vi "Retrieve and Scale Measurement.vi"(0 "private data":T1={"GTX2_CHANNEL register map"=refnum, "instruction target"=refnum, "channel measure state"=enum."Uninitialized", "in DFE mode?"=FALSE, "prescale"=0, "rx internal data width"=enum."32 Bit", "active point"={"horizontal offset"=0, "vertical offset"=0}, "ut sign"=enum."Positive", "positive counts"={"sample count"=0, "error count"=0}, "negative counts"={"sample count"=0, "error count"=0}}, 11 "error in":errorcluster) -> (4 "private data out":T1={"GTX2_CHANNEL register map"=refnum, "instruction target"=refnum, "channel measure state"=enum."Uninitialized", "in DFE mode?"=FALSE, "prescale"=0, "rx internal data width"=enum."32 Bit", "active point"={"horizontal offset"=0, "vertical offset"=0}, "ut sign"=enum."Positive", "positive counts"={"sample count"=0, "error count"=0}, "negative counts"={"sample count"=0, "error count"=0}}, 6 "bit error ratio":dbl, 8 "sample count":u64, 10 "error count":u64, 15 "error out":errorcluster)   [LabVIEW 2015, in "niHighSpeedSerial Eye Scan Single Point v1 Host.lvclass"]
doc: "Retrieves the saved <b>sample count(s)</b> and <b>error count(s)</b>, scales the <b>sample count(s)</b>, and computes the <b>bit error rate</b>.\n\n<B>Input Parameters</B>\n\n<B>private data</B> is the class private data input into the VI.\n\n<B>private data.GTX2_CHANNEL register map</B> is the GTX2 Channel register map to use.\n\n<B>private data.instruction target</B> is the instruction target to use when communicating with the FPGA.\n\n<B>private data.channel measure state</B> maintains the internal state of the Eye Scan Single Point class.\nenum values: Uninitialized,Initialized,Ready,Request,Wait,Read,Process,Finished\n\n<B>private data.in DFE mode?</B> is true if Eye Scan is configured for DFE Equalization Mode.\n\n<B>private data.prescale</B> controls scaling of the sample count in order to keep the sample count and error count within reasonable precision.\n\n<B>private data.receiver data width</B> is the data width (in bits) of the receiver lane.\nenum values: 16 Bit,20 Bit,32 Bit,40 Bit\n\n<B>private data.active point</B> is the point currently being sampled for errors using Eye Scan.\n\n<B>private data.active point.horizontal offset</B> is the horizontal offset of the active point.\n\n<B>private data.active point.vertical offset</B> is the vertical offset of the active point.\n\n<B>private data.ut sign</B> The untapped threshold sign (positive or negative) currently configured on the point being measured.\nPositive is used when in DFE or LPM Equalization Mode, while Negative is only used in DFE Equalization Mode.\n\n<B>private data.positive counts</B> contains the number of sample and error counts measured using the positive UT Sign.\n\n<B>private data.positive counts.sample count</B> is the positive sample count when using DFE mode, or the entire sample count when using LPM mode.\n\n<B>private data.positive counts.error count</B> is the positive error count when using DFE mode, or the entire error count when using LPM mode.\n\n<B>private data.negative counts</B> contains the number of sample and error counts measured using the negative UT Sign.\n\n<B>private data.negative counts.sample count</B> is the negative sample count when using DFE mode, or unused when using LPM mode.\n\n<B>private data.negative counts.error count</B> is the negative error count when using DFE mode, or unused when using LPM mode.\n\n<B>error in</B> describes error conditions that occur before this node runs. This input provides standard 'error in' functionality.\n\n<B>Output Parameters</B>\n\n<B>private data out</B> is the class private data output from the VI.\n\n<B>private data out.GTX2_CHANNEL register map</B> is the register map to use which represents the GTX2 Channel.\n\n<B>private data out.instruction target</B> is the instruction target to use when communicating with the FPGA.\n\n<B>private data out.channel measure state</B> maintains the internal state of the Eye Scan Single Point class.\nenum values: Uninitialized,Initialized,Ready,Request,Wait,Read,Process,Finished\n\n<B>private data out.in DFE mode?</B> is true if Eye Scan is configured for DFE Equalization Mode.\n\n<B>private data out.prescale</B> controls scaling of the sample count in order to keep the sample count and error count within reasonable precision.\n\n<B>private data out.receiver data width</B> is the data width (in bits) of the receiver lane.\nenum values: 16 Bit,20 Bit,32 Bit,40 Bit\n\n<B>private data out.active point</B> is the point currently being sampled for errors using Eye Scan.\n\n<B>private data out.active point.horizontal offset</B> is the horizontal offset of the active point.\n\n<B>private data out.active point.vertical offset</B> is the vertical offset of the active point.\n\n<B>private data out.ut sign</B> contains the number of sample and error counts measured using the positive UT Sign.\nenum values: Positive,Negative\n\n<B>private data out.positive counts</B> contains the number of sample and error counts measured using the positive UT Sign.\n\n<B>private data out.positive counts.sample count</B> is the positive sample count when using DFE mode, or the entire sample count when using LPM mode.\n\n<B>private data out.positive counts.error count</B> is the positive error count when using DFE mode, or the entire error count when using LPM mode.\n\n<B>private data out.negative counts</B> contains the number of sample and error counts measured using the negative UT Sign.\n\n<B>private data out.negative counts.sample count</B> is the negative sample count when using DFE mode, or the entire sample count when using LPM mode.\n\n<B>private data out.negative counts.error count</B> is the negative error count when using DFE mode, or the entire error count when using LPM mode.\n\n<B>bit error rate</B> is the calculated statistical bit error rate based on the number of error counts and sample counts received.\n\n<B>sample count</B> is the number of samples that have been measured on this point.\n\n<B>error count</B> is the number of errors that have been measured on this point.\n\n<B>error out</B> contains error information. This output provides standard 'error out' functionality."
uses:
  <instrlib>/niHighSpeedSerial/Eye Scan/v1/Host/Impl/Single Point/niHighSpeedSerial Eye Scan Single Point v1 Host.lvclass
  <instrlib>/niHighSpeedSerial/Eye Scan/v1/Host/Impl/Single Point/Private/Private Data.ctl
  <instrlib>/niHighSpeedSerial/Register Maps/Xilinx/v1/Host/GTX2_CHANNEL v1 Host.llb/GTX2_CHANNEL Register Map.lvclass
  <instrlib>/_niInstr/Instruction Framework/v1/Host/Instruction Target/niInstr Instruction Target v1 Host.lvclass
  <instrlib>/niHighSpeedSerial/Eye Scan/v1/Host/Impl/Single Point/Private/Channel Measure State.ctl
  <instrlib>/niHighSpeedSerial/Eye Scan/v1/Host/Common/Public/Data Width.ctl
  <instrlib>/niHighSpeedSerial/Eye Scan/v1/Host/Common/Public/Point Offsets.ctl
  <instrlib>/niHighSpeedSerial/Register Maps/Xilinx/v1/Host/GTX2_CHANNEL v1 Host.llb/ESVertOffsetSign.ctl
  <instrlib>/niHighSpeedSerial/Eye Scan/v1/Host/Impl/Single Point/Private/Counts.ctl
  <instrlib>/niHighSpeedSerial/Eye Scan/v1/Host/Common/niHighSpeedSerial Eye Scan Common v1 Host.lvlib
  <instrlib>/niHighSpeedSerial/Register Maps/Xilinx/v1/Host/GTX2_CHANNEL v1 Host.llb/GTX2_CHANNEL v1 Host.lvlib
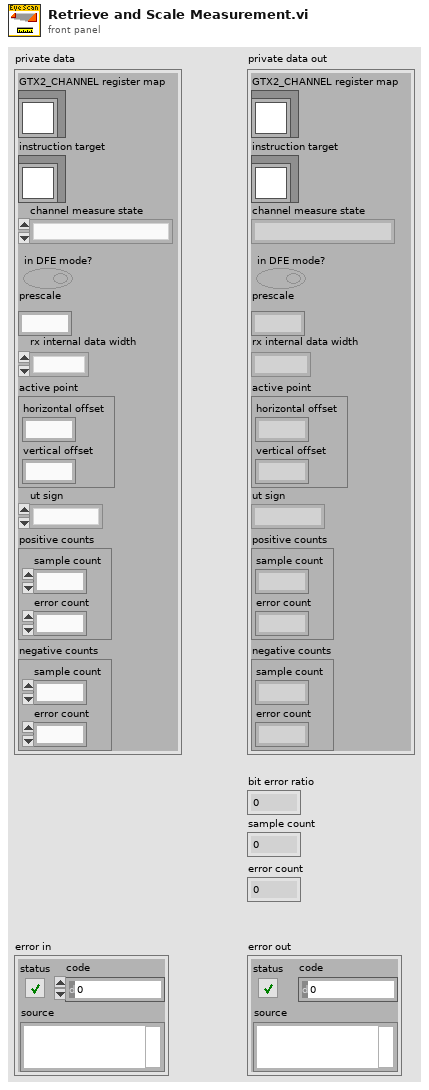
[diagram p1: front panel]
types:
  T1 = typedef "niHighSpeedSerial Eye Scan Single Point v1 Host.lvclass/Private Data.ctl" = cluster{"GTX2_CHANNEL register map":refnum<class "GTX2_CHANNEL Register Map.lvclass">, "instruction target":refnum<class "niInstr Instruction Target v1 Host.lvclass">, "channel measure state":T2, "in DFE mode?":bool, "prescale":u8, "rx internal data width":T3, "active point":T4, "ut sign":T5, "positive counts":T6, "negative counts":T6}
  T2 = typedef "niHighSpeedSerial Eye Scan Single Point v1 Host.lvclass/Channel Measure State.ctl" = enum16{"Uninitialized", "Initialized", "Ready", "Request", "Wait", "Read", "Process", "Finished"}
  T3 = typedef "niHighSpeedSerial Eye Scan Common v1 Host.lvlib/Data Width.ctl" = enum16{"16 Bit", "20 Bit", "32 Bit", "40 Bit"}
  T4 = typedef "niHighSpeedSerial Eye Scan Common v1 Host.lvlib/Point Offsets.ctl" = cluster{"horizontal offset":i16, "vertical offset":i8}
  T5 = typedef "GTX2_CHANNEL v1 Host.lvlib/ESVertOffsetSign.ctl" = enum8{"Positive", "Negative"}
  T6 = typedef "niHighSpeedSerial Eye Scan Single Point v1 Host.lvclass/Counts.ctl" = cluster{"sample count":u64, "error count":u16}
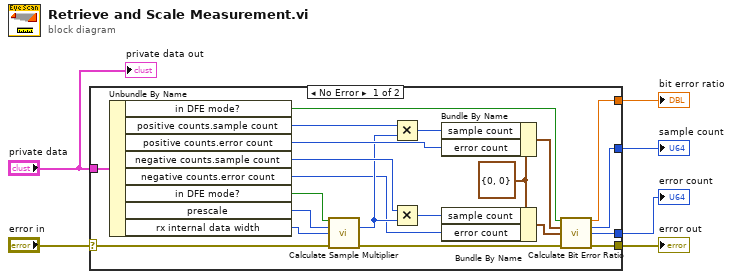
[diagram p0: block diagram]
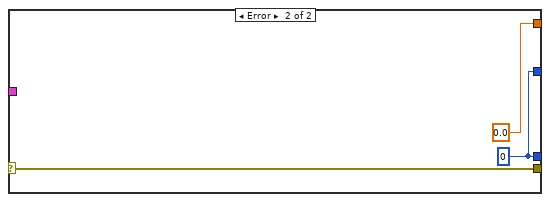
[diagram p2: hidden frame]
diagram:
  n1 = case shown="No Error" "error in" {
    selector: "error in" -> [w27 w30]
    tunnel: [w16 w30] -> w5
    tunnel: "private data" -> [w26 _]
    tunnel: [w12 0.0 ("bit error ratio")] -> w4
    tunnel: [w11 w28] -> w3
    tunnel: [w10 w28] -> w2
    frame No Error {
      w18 = T6 {"sample count"=0, "error count"=0} ("counts")
      n2 = Unbundle By Name(w26) -> ("in DFE mode?"=w13:bool, "positive counts.sample count"=w25:u64, "positive counts.error count"=w23:u16, "negative counts.sample count"=w21:u64, "negative counts.error count"=w19:u16, "in DFE mode?"=w9:bool, "prescale"=w8:u8, "rx internal data width"=w7:T3)
      n3 = call <instrlib>:"Calculate Sample Multiplier.vi"("in DFE mode?"=w9, "prescale"=w8, "receiver data width"=w7, "error in"=w27) -> ("sample multiplier"=w20:u64, "error out"=w17:errorcluster)  [unwired: 9 in, 1 out]
      n4 = Multiply(x=w25, y=w20) -> (x*y=w24:u64)
      n5 = Multiply(x=w21, y=w20) -> (x*y=w22:u64)
      n6 = Bundle By Name(cluster=w18, "sample count"=w24, "error count"=w23) -> (w15:T6)
      n7 = Bundle By Name(cluster=w18, "sample count"=w22, "error count"=w19) -> (w14:T6)
      n8 = call <instrlib>:"Calculate Bit Error Ratio.vi"("in DFE mode?"=w13, "positive counts"=w15, "negative counts"=w14, "error in"=w17) -> ("bit error ratio"=w12:dbl, "sample count"=w10:u64, "error count"=w11:u64, "error out"=w16:errorcluster)  [unwired: 8 in]
    }
    frame Error {
      w28 = u64 0 ("sample count")
    }
  }
  "error out" <- w5
  "bit error ratio" <- w4
  "sample count" <- w2
  "error count" <- w3
  "private data out" <- "private data"
